vi "Host - Altimeter Data (SubVI).vi"(11 "Altimeter Data":string) -> (3 "altitute in meters":dbl)   [LabVIEW 2021]
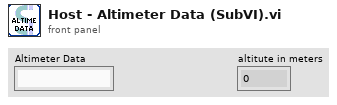
[diagram p1: front panel]
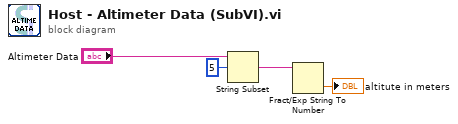
[diagram p0: block diagram]
diagram:
  n1 = String Subset(string="Altimeter Data", offset (0)=5) -> (substring=w3:string)  [unwired: 1 out]
  n2 = Fract/Exp String To Number(string=w3) -> (number=→"altitute in meters":dbl)  [unwired: 4 out]
